vi "List UIPs Recursive.vi"(11 "Plugin Folder Path":path) -> (2 "UIPs":refnum<class "UIP.lvclass">[](array[class]), 3 "Plugin Folder Path Out":path)   [LabVIEW 2015, in "UIM.lvclass"]
doc: "Traverses a location for UIP plugins and returns them initialized to default values. This can be used to point to your folder of plugins and load them easily.\n\n<b> NOTE </b> - This is a recursive function traversing the folder structure. Use with caution."
uses:
  UIM.lvclass
  UIP/UIP.lvclass
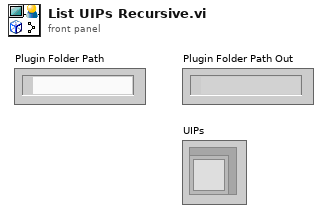
[diagram p1: front panel]
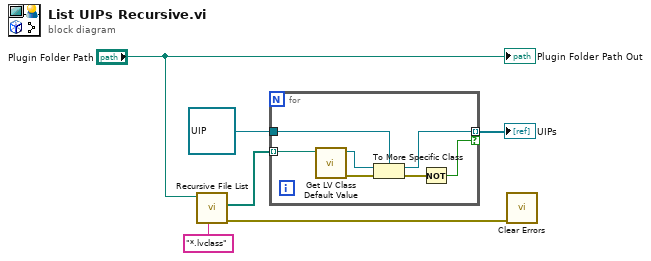
[diagram p0: block diagram]
diagram:
  n1 = call <vilib>:"Recursive File List.vi"("pattern"="*.lvclass", "Folder Path"="Plugin Folder Path") -> ("error out"=w3:errorcluster, "All Files in Dir"=w5:path[])  [unwired: 5 in, 3 out]
  n2 = for {
    tunnel: w5 -> [w13] mode=indexing
    tunnel: [w10] -> w2 mode=indexing if=w8
    tunnel: refnum<class "UIP.lvclass"> refnum ("UIP") -> [w7]
    n3 = call <vilib>:"Get LV Class Default Value.vi"("class path"=w13) -> ("error out"=w12:errorcluster, "object"=w11:refnum<class>)  [unwired: 9 in]
    n4 = To More Specific Class(target class=w7, reference=w11, error in=w12) -> (specific class reference=w10:refnum<class "UIP.lvclass">, error out=w9:errorcluster)
    n5 = Not(x=w9) -> (.not. x?=w8:bool)
  }
  "UIPs" <- w2
  n6 = call <vilib>:"Clear Errors.vi"("error in (no error)"=w3) -> ()  [unwired: 5 in, 2 out]
  "Plugin Folder Path Out" <- "Plugin Folder Path"
